vi "Disconnect.vi"(8 "error in (no error)":errorcluster, 11 "PXIe5413 in":refnum<class "PXIe5413.lvclass">) -> (0 "error out":errorcluster, 3 "PXIe5413 out":refnum<class "PXIe5413.lvclass">)   [LabVIEW 2018, in "PXIe5413.lvlib" / "PXIe5413.lvclass"]
uses:
  PXIe5413.lvclass
  PPLs/Function Generator/Parent/Function Generator.lvlibp/Function Generator.lvclass
  C:/Projects/LabVIEW/PPLs/Function Generator/Parent/Function Generator.lvlibp/Function Generator.lvclass
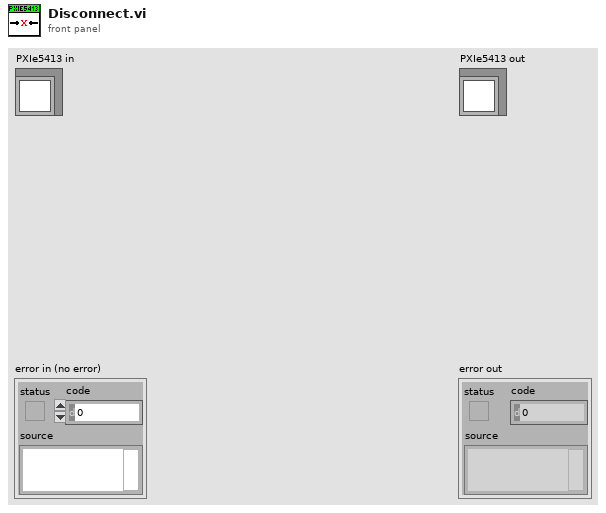
[diagram p1: front panel]
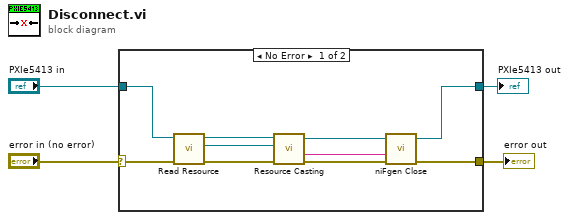
[diagram p0: block diagram]
diagram:
  n1 = case shown="No Error" "error in (no error)" {
    selector: "error in (no error)" -> [w13 w15]
    tunnel: [w6 w15] -> w3
    tunnel: [w7 w14] -> w2
    tunnel: "PXIe5413 in" -> [w12 w14]
    frame No Error {
      n2 = call "Read Resource.vi"("error in (no error)"=w13, "Function Generator in"=w12) -> ("error out"=w11:errorcluster, "Resource"=w5:refnum<visa-resource-name>, "Function Generator out"=w10:refnum<class "PXIe5413.lvclass">)  [unwired: 7 in]
      n3 = call "Resource Casting.vi"("error in (no error)"=w11, "VISA Resource In"=w5, "PXIe5413 in"=w10) -> ("error out"=w8:errorcluster, "Casted Resource"=w9:string, "PXIe5413 out"=w7:refnum<class "PXIe5413.lvclass">)  [unwired: 6 in]
      n4 = call <instrlib>:"niFgen Close.vi"("error in (no error)"=w8, "Instrument Handle"=w9) -> ("error out"=w6:errorcluster)  [unwired: 9 in]
    }
    frame Error {
    }
  }
  "error out" <- w3
  "PXIe5413 out" <- w2
